vi "Apply Motor Config Obj.vi"(8 "error in (no error)":errorcluster, 10 "Motor Config Obj":refnum<class "Motor Configuration.lvclass">, 11 "VacuumLine Configuration in":refnum<class "VacuumLine Configuration.lvclass">) -> (0 "error out":errorcluster, 3 "VacuumLine Configuration out":refnum<class "VacuumLine Configuration.lvclass">)   [LabVIEW 2016, in "Hardware.lvlib" / "VacuumLine.lvlib" / "VacuumLine Configuration.lvclass"]
uses:
  <userlib>/Common Components/Hardware/Abstract System/VacuumLine/VacuumLine Config/VacuumLine Configuration.lvclass
  <userlib>/Common Components/Hardware/Motor/Motor Config/Motor Configuration.lvclass
  <userlib>/Common Components/Hardware/Abstract System/VacuumLine/VacuumLine Config/VacuumLine Configuration.lvclass/VacuumLine Configuration.ctl
  <userlib>/Common Components/Hardware/Abstract System/VacuumLine/VacuumLine/VacuumLine.lvclass/VacuumLine.ctl
  <userlib>/Common Components/Hardware/Abstract System/VacuumLine/VacuumLine/VacuumLine.lvclass
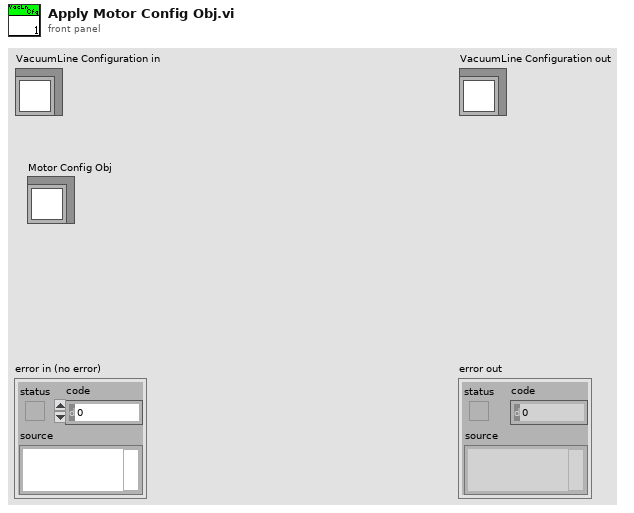
[diagram p1: front panel]
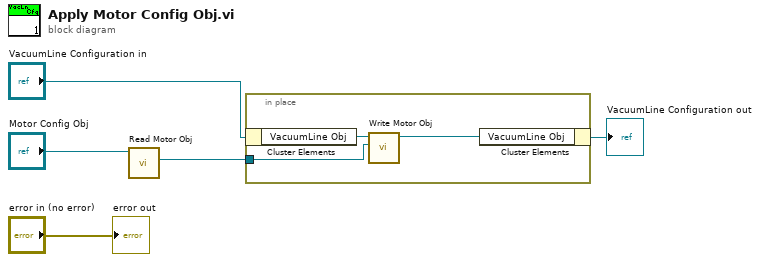
[diagram p0: block diagram]
diagram:
  n1 = call <userlib>:"Read Motor Obj.vi"("Motor Configuration in"="Motor Config Obj") -> ("Hardware.lvlib:Motor.lvlib:Motor.lvclass"=w3:refnum<class "Motor.lvclass">)  [unwired: 8 in, 2 out]
  n2 = in-place {
    in-place-border: w3 -> [w8]
    n3 = in-place-cluster #1("VacuumLine Configuration in") -> ("VacuumLine Obj"=w7:refnum<class "VacuumLine.lvclass">)
    n4 = call <userlib>:"Write Motor Obj.vi"("Hardware.lvlib:Motor.lvlib:Motor.lvclass"=w8, "VacuumLine in"=w7) -> ("VacuumLine out"=w6:refnum<class "VacuumLine.lvclass">)  [unwired: 8 in, 1 out]
    n5 = in-place-cluster #1("VacuumLine Obj"=w6) -> (→"VacuumLine Configuration out":refnum<class "VacuumLine Configuration.lvclass">)
  }
  "error out" <- "error in (no error)"
